vi "P3.1.vi"() -> ()   [LabVIEW 2020]
uses:
  <vilib>/Analysis/2dsp.llb/Real FFT.vi
  <vilib>/Analysis/NI_AALPro.lvlib
panel:
  out "X":dbl[](array[numeric])
  out "FFT {X}":cdb[](array[numeric])
  in  "FFT size":i32=-1
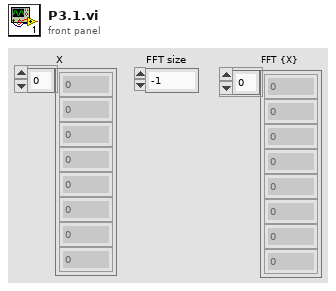
[diagram p1: front panel]
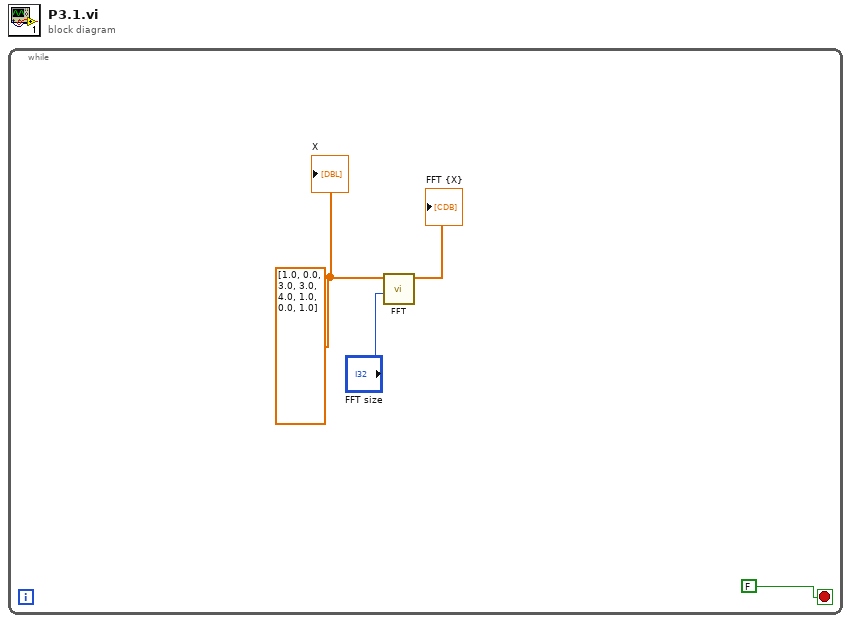
[diagram p0: block diagram]
diagram:
  n1 = while {
    stop <- FALSE ("stop") stop-if-true
    w4 = dbl[] [1.0, 0.0, 3.0, 3.0, 4.0, 1.0, 0.0, 1.0] ("X")
    n2 = call-poly <vilib>:"FFT.vi"("FFT size"="FFT size", "X"=w4) -> ("FFT {X}"=→"FFT {X}":cdb[])  [unwired: 8 in, 1 out]
    "X" <- w4
  }
